vi "Enable Line Cycle Synchronization.vi"(8 "error in (no error)":errorcluster, 10 "Enable Line Cycle Synchronization (T: Enable)":bool=TRUE, 11 "VISA resource name":refnum<visa-resource-name>) -> (0 "error out":errorcluster, 3 "VISA resource name out":refnum<visa-resource-name>)   [LabVIEW 2011, in "Keithley 2182.lvlib"]
doc: "Enables or disables instrument's Line Cycle Synchronization feature.\n\nWhen enabled, A/D conversions are synchronized with the power line frequency. This\nreduces noise at the expense of speed. Line cycle synchronization (LSYNC) is not available for\nintegration rates <1 PLC, regardless of the LSYNC setting."
uses:
  Keithley 2182.lvlib
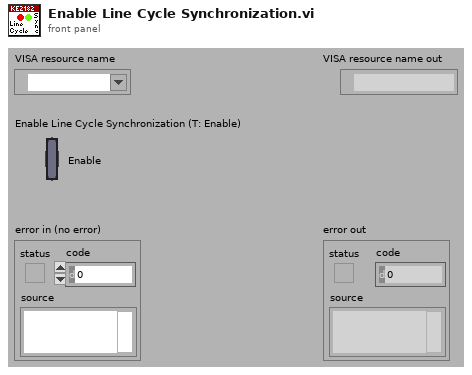
[diagram p1: front panel]
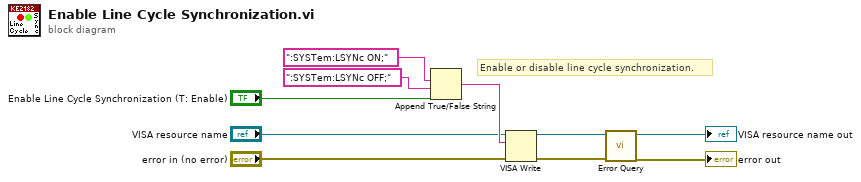
[diagram p0: block diagram]
diagram:
  # "Enable or disable line cycle synchronization."
  n1 = Append True/False String(1:"Enable Line Cycle Synchronization (T: Enable)", 2:":SYSTem:LSYNc OFF;", 3:":SYSTem:LSYNc ON;") -> (0:w7:string)  [unwired: 1 in]
  n2 = VISA Write(VISA resource name="VISA resource name", write buffer=w7, error in (no error)="error in (no error)") -> (VISA resource name out=w4:refnum<visa-resource-name>, error out=w3:errorcluster)  [unwired: 1 out]
  n3 = call "Error Query.vi"("error in (no error)"=w3, "VISA resource name"=w4) -> ("error out"=→"error out":errorcluster, "VISA resource name out"=→"VISA resource name out":refnum<visa-resource-name>)  [unwired: 6 in, 2 out]
